vi "Convert2ValidCylinderCalibrParams.vi"(1 "CylinderCalibrNew in":T1 {"ZsignalHeightDependence (1/nm)" format="%.4e"}) -> (0 "CylinderCalibrNew out":T1 {"ZsignalHeightDependence (1/nm)" format="%.4e"})   [LabVIEW 2020, in "Initialization.lvlib" / "FileManagement.lvlib"]
uses:
  FileManagement.lvlib
  CylinderCalibrNew.ctl
  Initialization.lvlib
panel:
  # "Convert the calibration to effective values"
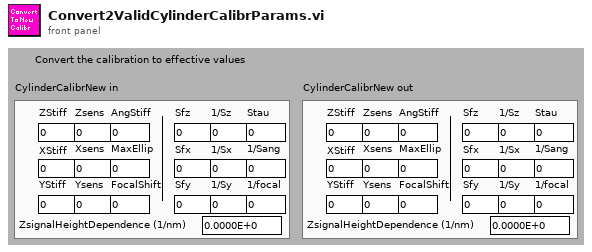
[diagram p1: front panel]
types:
  T1 = typedef "Initialization.lvlib/CylinderCalibrNew.ctl" = cluster{"ZStiff":dbl, "Zsens":dbl, "AngStiff":dbl, "XStiff":dbl, "Xsens":dbl, "MaxEllip":dbl, "YStiff":dbl, "Ysens":dbl, "FocalShift":dbl, "Sfz":dbl, "1/Sz":dbl, "Stau":dbl, "Sfx":dbl, "1/Sx":dbl, "1/Sang":dbl, "Sfy":dbl, "1/Sy":dbl, "1/focal":dbl, "ZsignalHeightDependence (1/nm)":dbl}
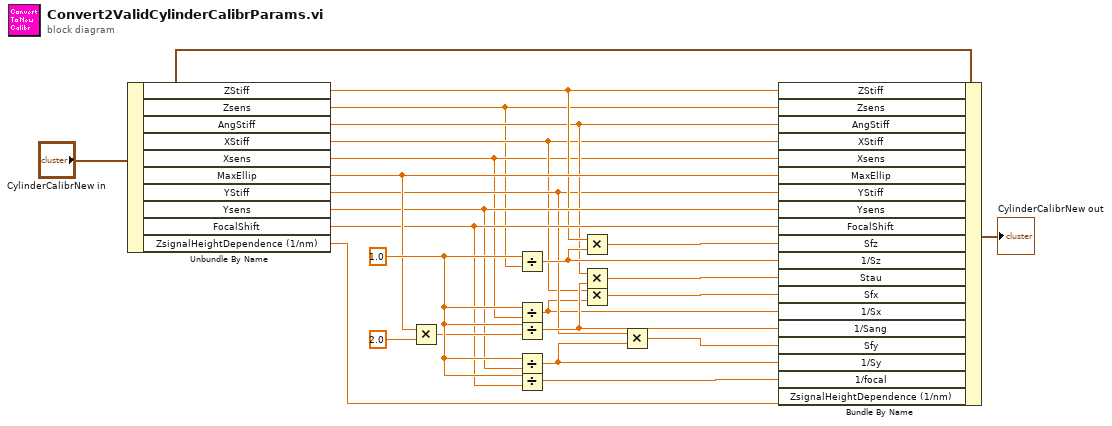
[diagram p0: block diagram]
diagram:
  w22 = 1.0 ("x")
  n1 = Unbundle By Name("CylinderCalibrNew in") -> ("ZStiff"=w14:dbl, "Zsens"=w2:dbl, "AngStiff"=w11:dbl, "XStiff"=w5:dbl, "Xsens"=w3:dbl, "MaxEllip"=w20:dbl, "YStiff"=w8:dbl, "Ysens"=w17:dbl, "FocalShift"=w18:dbl, "ZsignalHeightDependence (1/nm)"=w1:dbl)
  n2 = Multiply(x=w20, y=2.0 ("x")) -> (x*y=w21:dbl)
  n3 = Divide(x=w22, y=w2) -> (x/y=w15:dbl)
  n4 = Divide(x=w22, y=w3) -> (x/y=w6:dbl)
  n5 = Divide(x=w22, y=w21) -> (x/y=w12:dbl)
  n6 = Divide(x=w22, y=w17) -> (x/y=w9:dbl)
  n7 = Divide(x=w22, y=w18) -> (x/y=w19:dbl)
  n8 = Multiply(x=w14, y=w15) -> (x*y=w16:dbl)
  n9 = Multiply(x=w11, y=w12) -> (x*y=w13:dbl)
  n10 = Multiply(x=w5, y=w6) -> (x*y=w7:dbl)
  n11 = Multiply(x=w8, y=w9) -> (x*y=w10:dbl)
  n12 = Bundle By Name(cluster="CylinderCalibrNew in", "ZStiff"=w14, "Zsens"=w2, "AngStiff"=w11, "XStiff"=w5, "Xsens"=w3, "MaxEllip"=w20, "YStiff"=w8, "Ysens"=w17, "FocalShift"=w18, "Sfz"=w16, "1/Sz"=w15, "Stau"=w13, "Sfx"=w7, "1/Sx"=w6, "1/Sang"=w12, "Sfy"=w10, "1/Sy"=w9, "1/focal"=w19, "ZsignalHeightDependence (1/nm)"=w1) -> (→"CylinderCalibrNew out":T1)
